vi "SetPWM.vi"(8 "error in (no error)":errorcluster, 9 "Value":u16, 10 "Led num":u8, 11 "Motorshield in":refnum<class "Motorshield.lvclass">) -> (0 "error out":errorcluster, 3 "Motorshield out":refnum<class "Motorshield.lvclass">)   [LabVIEW 2022 SP3, in "Motorshield.lvlib" / "Motorshield.lvclass"]
uses:
  Motorshield.lvclass
  Motorshield.lvclass/Motorshield.ctl
  pca985/PCA/PCA.lvclass
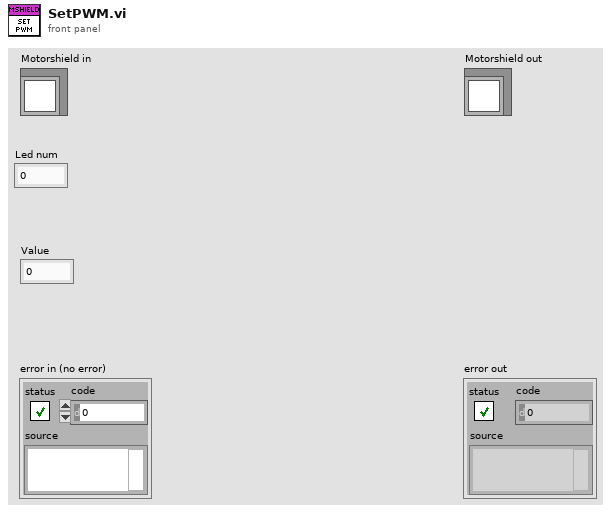
[diagram p1: front panel]
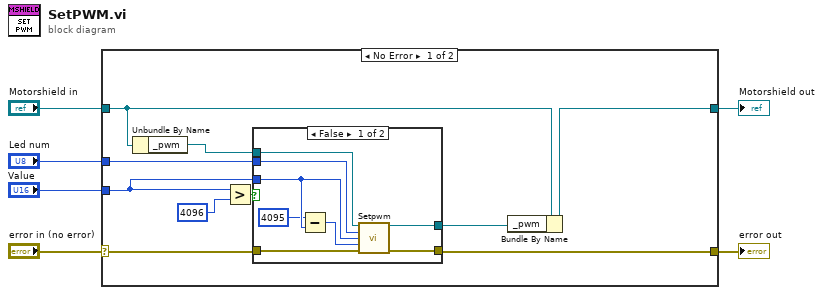
[diagram p0: block diagram]
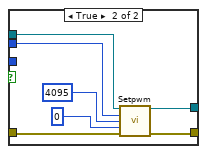
[diagram p2: hidden frame]
diagram:
  n1 = case shown="No Error" "error in (no error)" {
    selector: "error in (no error)" -> [w16 w33]
    tunnel: [w15 w33] -> w5
    tunnel: [w8 w32] -> w3
    tunnel: "Motorshield in" -> [w14 w32]
    tunnel: "Led num" -> [w12 _]
    tunnel: "Value" -> [w9 _]
    frame No Error {
      n2 = Unbundle By Name(w14) -> ("_pwm"=w13:refnum<class "PCA.lvclass">)
      n3 = Greater?(x=w9, y=4096) -> (0:w11:bool)
      n4 = case shown="False" w11 {
        tunnel: w16 -> [w24 w31]
        tunnel: [w23 w30] -> w15
        tunnel: w13 -> [w22 w29]
        tunnel: w12 -> [w21 w28]
        tunnel: w9 -> [w19 _]
        tunnel: [w20 w25] -> w7
        frame False {
          n5 = Subtract(x=u16 4095, y=w19) -> (x-y=w17:u16)
          n6 = call "Setpwm.vi"("PCA in"=w22, "Led num"=w21, "on"=w19, "off"=w17, "error in (no error)"=w24) -> ("PCA out"=w20:refnum<class "PCA.lvclass">, "error out"=w23:errorcluster)  [unwired: 8 in, 1 out]
        }
        frame True {
          n7 = call "Setpwm.vi"("PCA in"=w29, "Led num"=w28, "on"=4095, "off"=0, "error in (no error)"=w31) -> ("PCA out"=w25:refnum<class "PCA.lvclass">, "error out"=w30:errorcluster)  [unwired: 8 in, 1 out]
        }
      }
      n8 = Bundle By Name(cluster=w14, "_pwm"=w7) -> (w8:refnum<class "Motorshield.lvclass">)
    }
    frame Error {
    }
  }
  "error out" <- w5
  "Motorshield out" <- w3
